vi "Passive Force Clamp-final-v2.vi"(4 "file name add to the end (height)":string="h300", 5 "feedback?":bool, 6 "X=T,Y=F":bool=TRUE, 7 "save?":bool, 8 "Set Force (pN)":dbl=45.0 format="%_8g", 9 "moving step size (um)":dbl=0.03, 10 "Auto Find":bool=TRUE, 11 "range (um)":dbl=2.0 format="%.3f") -> ()   [LabVIEW 2014]
uses:
  <vilib>/Analysis/baseanly.llb/Mean (DBL).vi
  Main-Stage-Based/(Global) Current handle and LaserPower_YCC.vi
  <vilib>/Analysis/NI_AALBase.lvlib
panel:
  in  "Tab Control 2":enum32{"Force", "Power"}(tab)
  in  "Intensity Control, 0~-7000 (mV)":dbl=-600.0 format="%_8g"
  out "Lower Pos (um)":dbl
  out "Upper Pos (um)":dbl
  in  "jump (nm)":dbl=195.0
  out "Jump to middle (um)":dbl
  out "Max QPD-Stage Pos (um)":dbl
  in  "lower set value":dbl=0.26
  out "target QPD (V)":dbl
  in  "Avg. time delay (ms)":dbl=20.0
  out "True Target position":dbl
  out "Record scan rate  (um/s)":dbl=2.0
  out "Laser Lock?":bool
  out "Center QPD yc (V)":dbl format="%0.2f"
  out "Sampling rate after filtering (Hz)":dbl
  in  "Who's Data":enum16{"YCC", "PYW", "LCH", "YYH"}(ring)
  out "Stage-QPD data":dbl[][](array[numeric])
  out "Now position (um)":dbl
  in  "Avg points":i32=320
  out "True rate?":bool
  out "Real initial position (um)":dbl format="%0.5f"
  out "Axis":i32
  in  "toward+ ?\nT=+, F=-":bool
  out "target position (um)":dbl
  in  "upper set value":dbl=0.34
  in  "stop":bool
  in  "Tab Control":T1(tab)
  out "XY Graph":T2(graph)
  in  "Set Target position?":bool
  in  "Custom choose?":bool
  out "Z-QPD":dbl(graph)
  out "Waveform Chart":dbl[](graph)
  out "XY Graph 2":T3(graph)
  out "XY Graph 3":T3(graph)
  in  "Sampling rate":dbl=32000.0
  # "pFC region: jump 170 to 220"
  # "20R-- 300mV"
  # "peak~350 nm\nfrom r = 400 to 500 nm"
  # "jump to r=450 nm"
  # "2.9um for had acted"
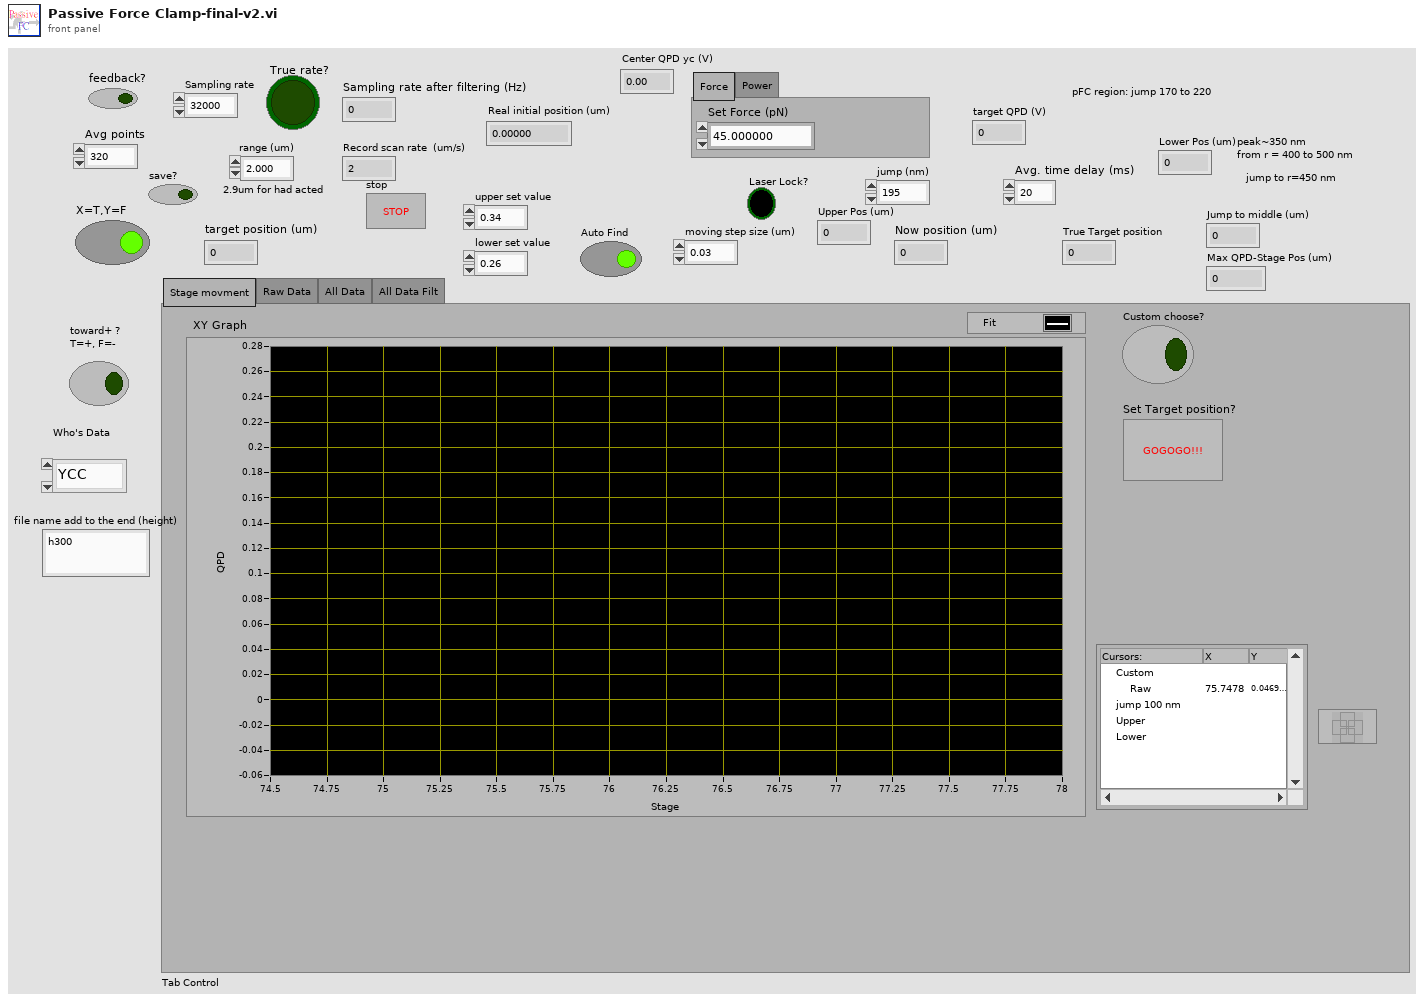
[diagram p1: front panel]
types:
  T1 = enum32{"Stage movment", "Raw Data", "All Data", "All Data Filt"}
  T2 = cluster{"Correct Unfolded Stage Array (um)":dbl[], "Filtered QPD Array":dbl[]}[]
  T3 = cluster{"Time Array (s)":dbl[], "Filtered QPD data":dbl[]}
  T4 = enum16{"Fixed-window avg", "Moving-window avg", "F+S-window avg", "S-G filter", "Fixed-window Median", "Moving-window Median "}
  T5 = cluster{"Correct Unfolded Stage Array (um)":dbl[], "Filtered QPD Array":dbl[]}
  T6 = cluster{"Time Array (s)":dbl[], "Filtered X":dbl[]}
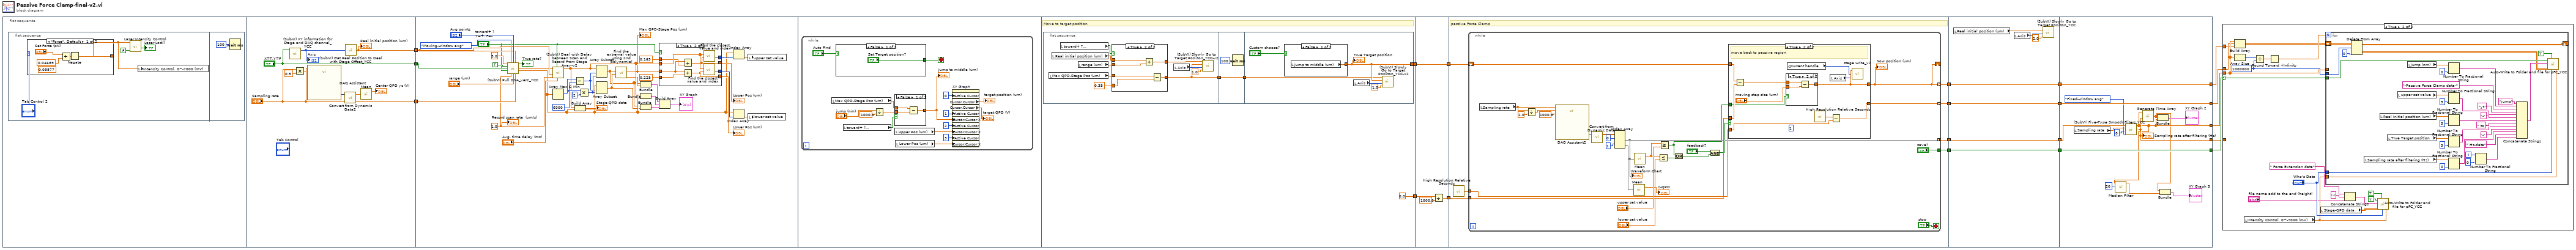
[diagram p0: block diagram]
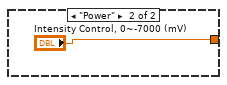
[diagram p3: hidden frame]
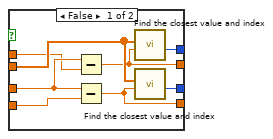
[diagram p4: hidden frame]
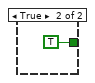
[diagram p5: hidden frame]
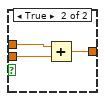
[diagram p6: hidden frame]
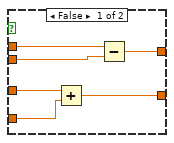
[diagram p7: hidden frame]
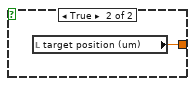
[diagram p8: hidden frame]
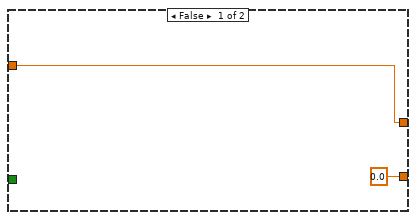
[diagram p9: hidden frame]
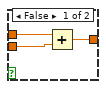
[diagram p10: hidden frame]
diagram:
  n1 = flat-sequence {
    tunnel: [w38] -> w17
    tunnel: ["X=T,Y=F"] -> w16
    tunnel: ["Sampling rate"] -> w5
    tunnel: w17 -> [w67]
    tunnel: w16 -> [w70]
    tunnel: w5 -> [w69]
    tunnel: [w119] -> w15
    tunnel: [0.0 ("Expect - Real move (nm)\nStage Offset\n+=more move\n-=less move")] -> w4
    tunnel: w15 -> [w154]
    tunnel: [w154] -> w14
    tunnel: [w152] -> w13
    tunnel: w4 -> [w151]
    tunnel: w14 -> [w158]
    tunnel: w13 -> [w157]
    tunnel: [w155] -> w11
    tunnel: [w160] -> w9
    tunnel: [w159] -> w7
    tunnel: [w156] -> w2
    tunnel: w11 -> [w213]
    tunnel: [w213] -> w10
    tunnel: w9 -> [w212]
    tunnel: [w212] -> w8
    tunnel: w7 -> [w211]
    tunnel: [w211] -> w6
    tunnel: [w207] -> w3
    tunnel: w2 -> [w207]
    tunnel: [w226] -> w18
    tunnel: [w227] -> w19
    tunnel: [w218] -> w20
    tunnel: w10 -> [w224]
    tunnel: w8 -> [w227]
    tunnel: w6 -> [w226]
    tunnel: [w220] -> w12
    tunnel: w3 -> [w225]
    tunnel: [w225] -> w1
    frame #0 {
      n2 = flat-sequence {
        frame #0 {
          n3 = case shown="\"Force\", Default" "Tab Control 2" {
            tunnel: [w27 "Intensity Control, 0~-7000 (mV)"] -> w21
            frame "Force", Default {
              (unwired) 0.03877 ("y")
              n4 = Divide(x="Set Force (pN)", y=0.04689) -> (x/y=w26:dbl)
              n5 = Negate(x=w26) -> (-x=w27:dbl)
            }
            frame "Power" {
            }
          }
          n6 = call "Laser Intensity Control.vi"("Close?"=FALSE, "Intensity Control, 0~-7000 (mV)"=w21) -> ("Laser Lock?"=→"Laser Lock?":bool)  [unwired: 5 in]
          n7 = local write "Intensity Control, 0~-7000 (mV)"(w21) -> ()
        }
        frame #1 {
          n8 = Wait (ms)(milliseconds to wait=u32 100) -> ()  [unwired: 1 out]
        }
      }
    }
    frame #1 {
      n9 = call "(SubVI) XY information for Stage and DAQ channel_YCC.vi"("T=X\nF=Y"="X=T,Y=F") -> ("Axis"=w39:i32)  [unwired: 3 in, 1 out]
      "Axis" <- w39
      n10 = Multiply(x="Sampling rate", y=0.5) -> (x*y=w34:dbl)
      n11 = call "DAQ Assistant"("rate"="Sampling rate", "number of samples"=w34) -> ("data"=w33:dynamicdata)  [unwired: 15 in, 2 out]
      n12 = call "Convert from Dynamic Data2"("Dynamic Data Type"=w33) -> ("Array"=w32:dbl[])  [unwired: 3 in]
      n13 = call "(SubVI) Get Real Position to Deal with Stage Offset_YCC.vi"("Axis"=w39) -> ("Real Current Commanded position (um)"=w38:dbl)  [unwired: 3 in, 1 out]
      "Real initial position (um)" <- w38
      n14 = call-poly <vilib>:"Mean.vi"("X"=w32) -> ("mean"=→"Center QPD yc (V)":dbl)  [unwired: 1 out]
    }
    frame #2 {
      w55 = 6000 ("y")
      w66 = 1.0 ("Record scan rate  (um/s)")
      n15 = call "(SubVI) Pull DNA_ver2_YCC.vi"("waiting time per point (ms)\nrange from 5ms to 0.167 ms"=5.0 ("waiting time per point (ms)\nrange from 5ms to 0.167 ms"), "Filter type"=T4."Moving-window avg", "Avg points"="Avg points", "Real initial position (um)"=w67, "Record?"=TRUE, "T=X\nF=Y"=w70, "Toward  ?\nT=+, F=-"="toward+ ?\nT=+, F=-", "Record scan rate  (um/s)"=w66, "range  (um)"="range (um)", "Sampling rate"=w69) -> ("True rate?"=→"True rate?":bool, "Filtered Stage Array"=w53:dbl[], "Filtered QPD Array"=w57:dbl[])  [unwired: 2 in, 1 out]
      n16 = call "(SubVI) Deal with Delay between Scan and Record From Stage Array-v2.vi"("Avg. time delay (ms)"="Avg. time delay (ms)", "Toward first ?\nT=+, F=-"="toward+ ?\nT=+, F=-", "Record scan rate  (um/s)"=w66, "Real initial position (um)"=w67, "Unfolded Stage Array (um)"=w53) -> ("Correct Unfolded Stage Array (um)"=w47:dbl[])  [unwired: 2 in, 2 out]
      n17 = Array Max & Min(array=w57) -> (max index (indices)=w56:i32)  [unwired: 3 out]
      n18 = Subtract(x=w56, y=w55) -> (x-y=w52:i32)
      n19 = Build Array(w47, w57) -> (→"Stage-QPD data":dbl[][])
      n20 = Multiply(x=w55, y=2) -> (x*y=w51:i32)
      n21 = Array Subset(array=w47, index=w52, length=w51) -> (w45:dbl[])
      n22 = Array Subset(array=w57, index=w52, length=w51) -> (w46:dbl[])
      n23 = call "Find the extremal value using 2nd polynomial.vi"("Y"=w46, "X"=w45) -> ("Best Polynomial Fit"=w44:dbl[], "Xm"=w42:dbl)  [unwired: 3 in, 1 out]
      "Max QPD-Stage Pos (um)" <- w42
      n24 = Bundle(w45, "Best Polynomial Fit"=w44) -> (w43:cluster{dbl[], "Best Polynomial Fit":dbl[]})  [unwired: 1 in]
      n25 = Bundle("Correct Unfolded Stage Array (um)"=w47, "Filtered QPD Array"=w57) -> (w50:T5)  [unwired: 1 in]
      n26 = Bundle(w45, w46) -> (w49:cluster{dbl[], dbl[]})  [unwired: 1 in]
      n27 = case shown="True" "toward+ ?\nT=+, F=-" {
        tunnel: w42 -> [w84 w92]
        tunnel: w47 -> [w83 w91]
        tunnel: [w82 w90] -> w63
        tunnel: [w81 w89] -> w62
        tunnel: 0.165 ("y") -> [w80 w88]
        tunnel: 0.225 ("y") -> [w79 w87]
        tunnel: [w78 w86] -> w59
        tunnel: [w77 w85] -> w58
        frame False {
          n28 = Subtract(x=w84, y=w80) -> (x-y=w78:dbl)
          n29 = Subtract(x=w84, y=w79) -> (x-y=w77:dbl)
          n30 = call "Find the closest value and index.vi"("Target Value"=w78, "Data"=w83) -> ("Closest Index of Value"=w82:i32)  [unwired: 4 in, 1 out]
          n31 = call "Find the closest value and index.vi"("Target Value"=w77, "Data"=w83) -> ("Closest Index of Value"=w81:i32)  [unwired: 4 in, 1 out]
        }
        frame True {
          n32 = Add(x=w92, y=w88) -> (x+y=w86:dbl)
          n33 = Add(x=w92, y=w87) -> (x+y=w85:dbl)
          n34 = call "Find the closest value and index.vi"("Target Value"=w86, "Data"=w91) -> ("Closest Index of Value"=w90:i32)  [unwired: 4 in, 1 out]
          n35 = call "Find the closest value and index.vi"("Target Value"=w85, "Data"=w91) -> ("Closest Index of Value"=w89:i32)  [unwired: 4 in, 1 out]
        }
      }
      "Upper Pos (um)" <- w59
      "Lower Pos (um)" <- w58
      n36 = Build Array(w43, w50, w49) -> (→"XY Graph":T2)
      n37 = Index Array(array=w57, index=w63) -> (element=w61:dbl)
      n38 = Index Array(array=w57, index=w62) -> (element=w60:dbl)
      n39 = local write "upper set value"(w61) -> ()
      n40 = local write "lower set value"(w60) -> ()
      "Record scan rate  (um/s)" <- w66
    }
    frame #3 {
      n41 = while {
        stop <- w106 stop-if-true
        n42 = local read "Max QPD-Stage Pos (um)"() -> (w103:dbl)
        n43 = case shown="False" "Auto Find" {
          tunnel: ["Set Target position?" TRUE] -> w106
          frame False {
          }
          frame True {
          }
        }
        n44 = local read "toward+ ?\nT=+, F=-"() -> (w101:bool)
        n45 = Divide(x="jump (nm)", y=1000.0) -> (x/y=w98:dbl)
        n46 = case shown="False" w101 {
          tunnel: w103 -> [w113 w116]
          tunnel: w98 -> [w112 w115]
          tunnel: [w111 w114] -> w102
          frame False {
            n47 = Subtract(x=w113, y=w112) -> (x-y=w111:dbl)
          }
          frame True {
            n48 = Add(x=w116, y=w115) -> (x+y=w114:dbl)
          }
        }
        "Jump to middle (um)" <- w102
        n49 = local read "Upper Pos (um)"() -> (w95:dbl)
        n50 = local read "Lower Pos (um)"() -> (w94:dbl)
        n51 = property on="XY Graph" class="XYGraph (strict)"("Active Cursor"=u32 0, "Active Cursor"=u32 1, "Cursor.Cursor X"=w102, "Active Cursor"=u32 2, "Cursor.Cursor X"=w95, "Active Cursor"=u32 3, "Cursor.Cursor X"=w94) -> ("Cursor.Cursor X"=→"target position (um)":dbl, "Cursor.Cursor Y"=→"target QPD (V)":dbl)  [unwired: 2 in, 2 out]
      }
    }
    frame #4 {
      # "Move to target position"
      n52 = flat-sequence {
        tunnel: [w122] -> w118
        tunnel: w118 -> [w143]
        tunnel: [w143] -> w117
        tunnel: [w145] -> w119
        tunnel: w117 -> [w144]
        frame #0 {
          n53 = local read "Max QPD-Stage Pos (um)"() -> (w123:dbl)
          n54 = local read "Real initial position (um)"() -> (w125:dbl)
          n55 = local read "toward+ ?\nT=+, F=-"() -> (w127:bool)
          n56 = local read "range (um)"() -> (w126:dbl)
          n57 = case shown="True" w127 {
            tunnel: w125 -> [w134 w141]
            tunnel: w126 -> [w133 w140]
            tunnel: [w135 w139] -> w124
            tunnel: w123 -> [w132 w138]
            tunnel: [w131 w137] -> w122
            tunnel: 0.35 ("scan rate  (um/s)") -> [w130 w136]
            frame False {
              n58 = Add(x=w132, y=w130) -> (x+y=w131:dbl)
              n59 = Subtract(x=w134, y=w133) -> (x-y=w135:dbl)
            }
            frame True {
              n60 = Add(x=w141, y=w140) -> (x+y=w139:dbl)
              n61 = Subtract(x=w138, y=w136) -> (x-y=w137:dbl)
            }
          }
          n62 = local read "Axis"() -> (w129:i32)
          n63 = call "(SubVI) Slowly Go to Target Posiiton_YCC-v2.vi"("scan rate  (um/s)"=1.0, "axis"=w129, "Target position (um)"=w122, "Now position (um)"=w124) -> ()  [unwired: 2 in, 2 out]
        }
        frame #1 {
          n64 = Wait (ms)(milliseconds to wait=u32 100) -> ()  [unwired: 1 out]
        }
        frame #2 {
          n65 = case shown="False" "Custom choose?" {
            tunnel: [w149 w150] -> w145
            frame False {
              n66 = local read "Jump to middle (um)"() -> (w149:dbl)
            }
            frame True {
              n67 = local read "target position (um)"() -> (w150:dbl)
            }
          }
          "True Target position" <- w145
          n68 = local read "Axis"() -> (w148:i32)
          n69 = call "(SubVI) Slowly Go to Target Posiiton_YCC-v2.vi"("scan rate  (um/s)"=1.0, "axis"=w148, "Target position (um)"=w145, "Now position (um)"=w144) -> ()  [unwired: 2 in, 2 out]
        }
      }
    }
    frame #5 {
      n70 = Divide(x=w151, y=1000.0) -> (x/y=w152:dbl)
    }
    frame #6 {
      # "passive Force Clamp"
      n71 = call <vilib>:"High Resolution Relative Seconds.vi"() -> ("relative seconds"=w161:dbl)
      n72 = while {
        tunnel: w161 -> [w184]
        tunnel: [w183] -> w160 mode=indexing
        tunnel: [w170] -> w155 mode=concatenating
        tunnel: ["save?"] -> w159
        shift-right: [w162] -> _
        shift-left: w158 -> [w174]
        tunnel: w157 -> [w175]
        tunnel: [w162] -> w156 mode=indexing
        stop <- "stop" stop-if-true
        n73 = local read "Sampling rate"() -> (w178:dbl)
        n74 = Divide(x=w178, y=2.0) -> (x/y=w176:dbl)
        n75 = call "DAQ Assistant2"("rate"=w178, "number of samples"=w176, "timeout (s)"=1000.0) -> ("data"=w181:dynamicdata)  [unwired: 13 in, 3 out]
        n76 = call "Convert from Dynamic Data"("Dynamic Data Type"=w181) -> ("Array"=w173:dbl[][])  [unwired: 3 in]
        n77 = Index Array(array=w173, index (row) #1=0 ("index (row)"), index (row) #2=1 ("index (row)")) -> (element #1=w170:dbl[], element #2=w169:dbl[])  [unwired: 2 in]
        "Waveform Chart" <- w170
        n78 = call-poly <vilib>:"Mean.vi"("X"=w169) -> ("mean"=→"Z-QPD":dbl)  [unwired: 1 out]
        n79 = call-poly <vilib>:"Mean.vi"("X"=w170) -> ("mean"=w186:dbl)  [unwired: 1 out]
        n80 = Less Or Equal?(x=w186, y="lower set value") -> (x <= y?=w165:bool)
        n81 = Greater Or Equal?(x=w186, y="upper set value") -> (x >= y?=w163:bool)
        n82 = Or(x=w163, y=w165) -> (x .or. y?=w164:bool)
        n83 = And(x="feedback?", y=w164) -> (x .and. y?=w166:bool)
        n84 = case shown="True" w166 {
          tunnel: w184 -> [_ w199]
          tunnel: [0.0 w197] -> w183
          tunnel: [w188 w196] -> w162
          tunnel: w175 -> [_ w194]
          tunnel: w174 -> [w188 w191]
          tunnel: w163 -> [_ w190]
          frame False {
          }
          frame True {
            (unwired) 1 ("read #")
            # "move back to passive region"
            n85 = Subtract(x=w191, y=w194) -> (x-y=w193:dbl)
            n86 = case shown="True" w190 {
              tunnel: "moving step size (um)" -> [w201 w206]
              tunnel: [w203 w205] -> w196
              tunnel: w193 -> [w202 w204]
              frame False {
                n87 = Add(x=w202, y=w201) -> (x+y=w203:dbl)
              }
              frame True {
                n88 = Subtract(x=w204, y=w206) -> (x-y=w205:dbl)
              }
            }
            n89 = global read "(Global) Current handle and LaserPower_YCC.vi" "Current handle"() -> (w192:i32)
            n90 = call <vilib>:"High Resolution Relative Seconds.vi"() -> ("relative seconds"=w198:dbl)
            n91 = local read "Axis"() -> (w195:i32)
            n92 = Subtract(x=w198, y=w199) -> (x-y=w197:dbl)
            n93 = call "stage write_v2.vi"("axis"=w195, "Incoming Handle"=w192, "position"=w196) -> ()  [unwired: 2 in, 1 out]
          }
        }
        "Now position (um)" <- w162
      }
    }
    frame #7 {
      n94 = local read "Real initial position (um)"() -> (w209:dbl)
      n95 = local read "Axis"() -> (w210:i32)
      n96 = call "(SubVI) Slowly Go to Target Posiiton_YCC.vi"("scan rate  (um/s)"=2.0, "axis"=w210, "Target position (um)"=w209) -> ()  [unwired: 1 in, 4 out]
    }
    frame #8 {
      n97 = local read "Sampling rate"() -> (w222:dbl)
      n98 = call "(SubVI) Five-Type Smooth Filters_YCC.vi"("Filter type"=T4."Fixed-window avg", "Avg points"=8, "Sampling rate (Hz)"=w222, "QPD data"=w224) -> ("Sampling rate after filtering (Hz)"=w220:dbl, "Filtered QPD data"=w218:dbl[])  [unwired: 1 in]
      "Sampling rate after filtering (Hz)" <- w220
      n99 = call <vilib>:"Median Filter.vi"("left rank"=20, "X"=w218) -> ("Filtered X"=w216:dbl[])  [unwired: 8 in, 1 out]
      n100 = call "Generate Time Array.vi"("Data rate (Hz)"=w220, "Data"=w218) -> ("Time Array (s)"=w217:dbl[])  [unwired: 4 in]
      n101 = Bundle("Time Array (s)"=w217, "Filtered QPD data"=w218) -> (→"XY Graph 2":T3)  [unwired: 1 in]
      n102 = Bundle("Time Array (s)"=w217, "Filtered X"=w216) -> (→"XY Graph 3":T6)  [unwired: 1 in]
    }
  }
  n103 = case shown="True" w18 {
    selector: w18 -> [_ w245]
    tunnel: w20 -> [_ w241]
    tunnel: w19 -> [_ w240]
    tunnel: w12 -> [_ _]
    tunnel: w1 -> [_ w228]
    frame False {
    }
    frame True {
      w238 = 1000000 ("y")
      n104 = Build Array(w241, w240, w228) -> (w239:dbl[][])
      n105 = Array Size(array=w241) -> (size(s)=w242:i32)
      n106 = local read "Intensity Control, 0~-7000 (mV)"() -> (w229:dbl)
      n107 = Divide(x=w242, y=w238) -> (x/y=w244:dbl)
      n108 = Round Toward +Infinity(x=w244) -> (ceil(x): smallest int >= x=w243:dbl)
      n109 = local read "Stage-QPD data"() -> (w237:dbl[][])
      n110 = for {
        N: w243 -> [_]
        tunnel: w241 -> [_]
        tunnel: w245 -> [w271]
        shift-right: [w257] -> _
        shift-left: w239 -> [w262]
        tunnel: w238 -> [w261]
        tunnel: "Who's Data" -> [w256]
        tunnel: w229 -> [w251]
        i -> [w269]
        n111 = Delete From Array(array=w262, length=w261, index (col)=0 ("index (row)")) -> (deleted portion=w259:dbl[][], array with subset deleted=w257:dbl[][])  [unwired: 1 in]
        n112 = local read "Sampling rate after filtering (Hz)"() -> (w270:dbl)
        n113 = local read "Real initial position (um)"() -> (w280:dbl)
        n114 = local read "True Target position"() -> (w277:dbl)
        n115 = local read "upper set value"() -> (w254:dbl)
        n116 = local read "jump (nm)"() -> (w249:dbl)
        n117 = Number To Fractional String(number=w249, precision (6)=i16 0) -> (F-format string=w246:string)  [unwired: 2 in]
        n118 = Number To Fractional String(number=w254, precision (6)=i16 5) -> (F-format string=w252:string)  [unwired: 2 in]
        n119 = Number To Fractional String(number=w280, precision (6)=i16 3) -> (F-format string=w276:string)  [unwired: 2 in]
        n120 = Number To Fractional String(number=w277, precision (6)=i16 3) -> (F-format string=w274:string)  [unwired: 2 in]
        n121 = Number To Fractional String(number=w270, precision (6)=i16 0) -> (F-format string=w265:string)  [unwired: 2 in]
        n122 = Number To Fractional String(number=w269, precision (6)=i16 0) -> (F-format string=w263:string)  [unwired: 2 in]
        n123 = Concatenate Strings("jump" ("string"), w246, "-Passive Force Clamp data-" ("prompt"), "yt " ("string"), w252, "-" ("string"), w276, " to " ("string"), w274, "-" ("string"), w265, " Hz-data" ("string"), w263) -> (w272:string)
        n124 = call "Auto-Write to Folder and file for pFC_YCC.vi"("Current PD (mV)"=w251, "Who's Data"=w256, "T=2D\nF=1D"=TRUE ("T=2D\nF=1D"), "2D data to be saved"=w259, "File name add to the end \n(height)"=w272, "Save?"=w271) -> ()  [unwired: 2 in, 2 out]
      }
      n125 = Concatenate Strings(" Force Extension data" ("prompt"), "-" ("string"), "file name add to the end (height)") -> (w230:string)
      n126 = call "Auto-Write to Folder and file for pFC_YCC.vi"("Current PD (mV)"=w229, "Who's Data"="Who's Data", "T=2D\nF=1D"=TRUE ("T=2D\nF=1D"), "2D data to be saved"=w237, "File name add to the end \n(height)"=w230, "Save?"=TRUE) -> ()  [unwired: 2 in, 2 out]
    }
  }
